vi "split.vi"(9 "Threshold":dbl, 10 "points in":cluster{"Line":cluster{"X":dbl, "Y":dbl}[]}) -> (2 "line out":cluster{"Line":cluster{"X":dbl, "Y":dbl}[]}[](array[cluster]))   [LabVIEW 2016]
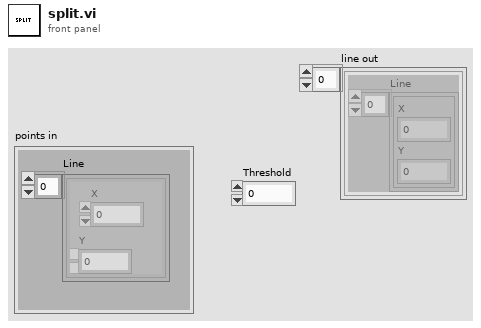
[diagram p1: front panel]
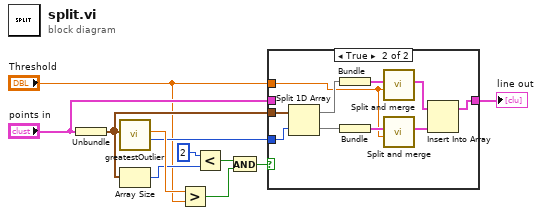
[diagram p0: block diagram]
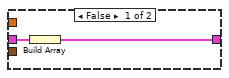
[diagram p2: hidden frame]
diagram:
  n1 = Unbundle("points in") -> ("Line"=w7:cluster{"X":dbl, "Y":dbl}[])
  n2 = call "greatestOutlier.vi"("line in"=w7) -> ("max index"=w8:i32, "max value"=w11:dbl)  [unwired: 9 in]
  n3 = Array Size(array=w7) -> (size(s)=w5:i32)
  n4 = Greater?(x=w11, y="Threshold") -> (0:w10:bool)
  n5 = Less?(x=2, y=w5) -> (x < y?=w3:bool)
  n6 = And(x=w3, y=w10) -> (x .and. y?=w9:bool)
  n7 = case shown="True" w9 {
    tunnel: w8 -> [_ w22]
    tunnel: w7 -> [_ w23]
    tunnel: [w12 w15] -> w6
    tunnel: "points in" -> [w13 _]
    tunnel: "Threshold" -> [_ w16]
    frame False {
      n8 = Build Array(w13) -> (w12:cluster{"Line":cluster{"X":dbl, "Y":dbl}[]}[])
    }
    frame True {
      n9 = Split 1D Array(array=w23, index=w22) -> (first subarray=w21:cluster{"X":dbl, "Y":dbl}[], second subarray=w14:cluster{"X":dbl, "Y":dbl}[])
      n10 = Bundle(w21) -> (w20:cluster{cluster{"X":dbl, "Y":dbl}[]})  [unwired: 1 in]
      n11 = Bundle(w14) -> (w19:cluster{cluster{"X":dbl, "Y":dbl}[]})  [unwired: 1 in]
      n12 = call "Split and merge.vi"("Threshold"=w16, "points in"=w20) -> ("line out"=w18:cluster{"Line":cluster{"X":dbl, "Y":dbl}[]}[])  [unwired: 9 in]
      n13 = call "Split and merge.vi"("Threshold"=w16, "points in"=w19) -> ("line out"=w17:cluster{"Line":cluster{"X":dbl, "Y":dbl}[]}[])  [unwired: 9 in]
      n14 = Insert Into Array(array=w18, new element=w17) -> (w15:cluster{"Line":cluster{"X":dbl, "Y":dbl}[]}[])  [unwired: 1 in]
    }
  }
  "line out" <- w6
